vi "PXI4072 NI-DMM Smoke Test (Custom).vi"() -> ()   [LabVIEW 2026]
uses:
  Drivers/PXI4072/Types/PXI4072 Settings.ctl
  <instrlib>/niDMM/nidmm.llb/niDMM Function.ctl
  <instrlib>/niDMM/nidmm.llb/niDMM Resolution in Digits.ctl
  Drivers/PXI4072/PXI4072.lvlib
panel:
  in  "Measurement Settings":T1={"Function"=enum."DC Volts", "Resolution in Digits"=5.5, "Range"=0.02} {"Range" format="%.2f"; "Resolution in Digits" items=["3 1/2"=3.5, "4 1/2"=4.5, "5 1/2"=5.5, "6 1/2"=6.5, "7 1/2"=7.5]}
  out "Measurement":dbl format="%.5f"
  in  "Resouce Name":refnum<k15> caption="Resource Name"
  in  "error in (no error)":errorcluster
  out "error out":errorcluster
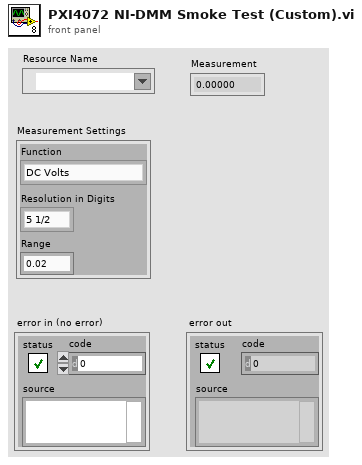
[diagram p1: front panel]
types:
  T1 = typedef "PXI4072.lvlib/PXI4072 Settings.ctl" = cluster{"Function":T2, "Resolution in Digits":T3, "Range":dbl}
  T2 = typedef "niDMM Function.ctl" = enum16{"DC Volts", "AC Volts", "DC Current", "AC Current", "2-wire Resistance", "4-wire Resistance", "Diode", "Frequency", "Period", "AC Volts DC Coupled", "Capacitance", "Inductance", "Temperature"}
  T3 = typedef "niDMM Resolution in Digits.ctl" = dbl
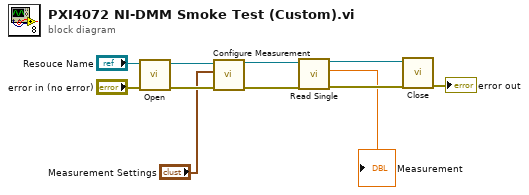
[diagram p0: block diagram]
diagram:
  n1 = call "Open.vi"("error in (no error)"="error in (no error)", "Resouce Name"="Resouce Name") -> ("error out"=w11:errorcluster, "Session Handle Out"=w3:refnum<k15>)  [unwired: 8 in]
  n2 = call "Configure Measurement.vi"("error in (no error)"=w11, "Measurement Settings"="Measurement Settings", "Session Handle"=w3) -> ("error out"=w10:errorcluster, "Session Handle Out"=w4:refnum<k15>)  [unwired: 7 in]
  n3 = call "Read Single.vi"("error in (no error)"=w10, "Session Handle"=w4) -> ("error out"=w9:errorcluster, "Measurement"=→"Measurement":dbl, "instrument handle out"=w5:refnum<k15>)  [unwired: 7 in]
  n4 = call "Close.vi"("error in (no error)"=w9, "Session Handle"=w5) -> ("error out"=→"error out":errorcluster)  [unwired: 9 in]
